vi "Send S&E Anotation message.vi"(2 "Send(T)":bool=TRUE, 7 "Annotation":string, 9 "error in (no error)":errorcluster, 12 "User(logged on)":string="Not Selected 1234", 13 "Elevated priority":bool) -> (6 "Loop ID out":u16, 10 "error out":errorcluster)   [LabVIEW 2011]
doc: "Put error message in the S&E Q. CAn also send if no error, debends exclusively on boolean in."
uses:
  emi Lib/System 01/0 - General/S&E reporting/Private/_emi_ S&E Message.ctl
  emi Lib/System 01/0 - General/S&E reporting/Private/_emi_ S&E Message type.ctl
  S&E Anotationtype.ctl
  emi Lib/System 01/0 - General/Private/_emi_GFV System ID.vi
panel:
  in  "Loc Sub ID":u16
  in  "Loop ID in(No Loop)":u16=9999
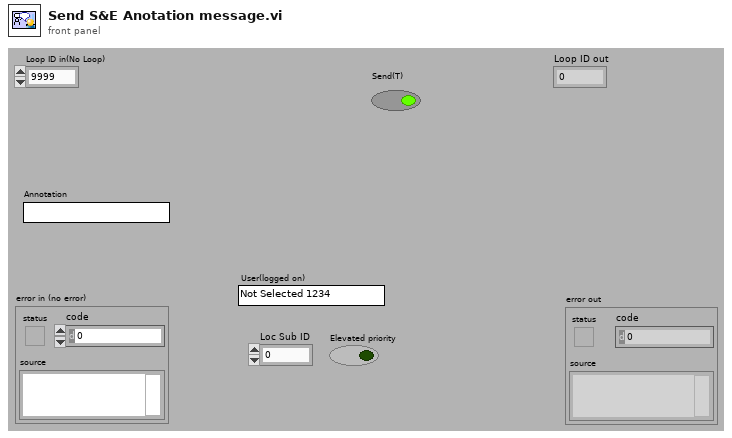
[diagram p1: front panel]
types:
  T1 = typedef "S&E Anotationtype.ctl" = cluster{"User":string, "Annotation":string}
  T2 = typedef "_emi_ S&E Message type.ctl" = enum16{"Error/Warning", "Note", "Debug", "Event", "Alarm Analog", "Alarm Digital", "Annotation"}
  T3 = typedef "_emi_ S&E Message.ctl" = cluster{"Type":T2, "Originate time":dbl, "System":u8, "Loop":u16, "Sub ID":u16, "Elevated priority":bool, "E&S Message content":variant}
  T4 = typedef "User Indikator.ctl" = cluster{"User Name":string, "Super User":T5}
  T5 = typedef "Super User bool indikator.ctl" = bool
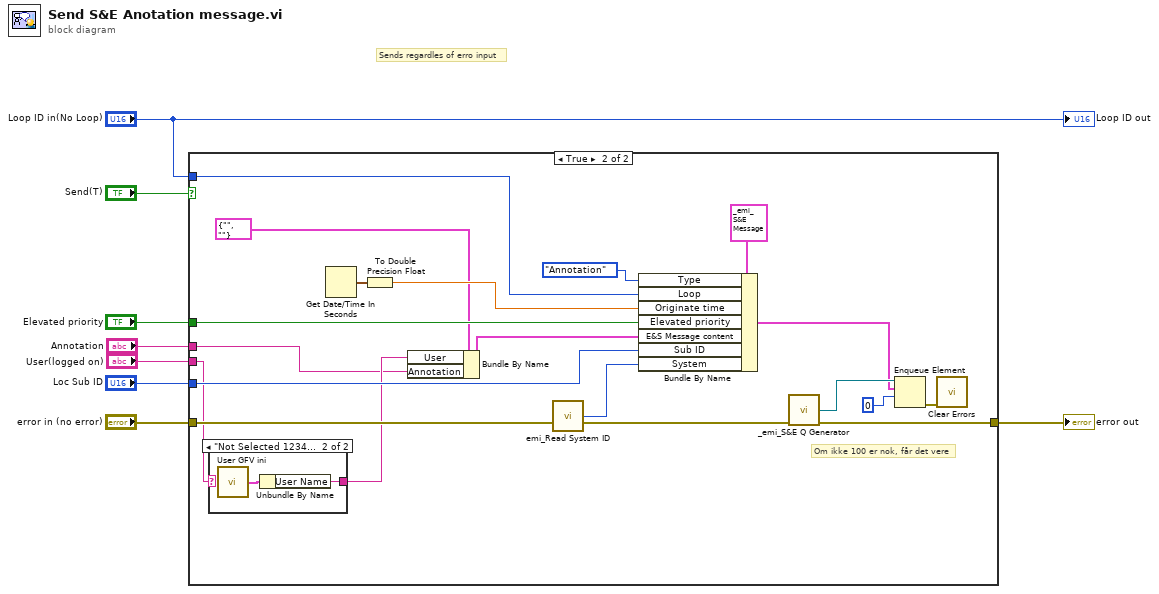
[diagram p0: block diagram]
diagram:
  # "Sends regardles of erro input"
  n1 = case shown="True" "Send(T)" {
    tunnel: "Loop ID in(No Loop)" -> [_ w25]
    tunnel: "Elevated priority" -> [_ w26]
    tunnel: "error in (no error)" -> [w9 w17]
    tunnel: [w9 w23] -> w5
    tunnel: "Loc Sub ID" -> [_ w19]
    tunnel: "User(logged on)" -> [_ w14]
    tunnel: "Annotation" -> [_ w10]
    frame False {
    }
    frame True {
      # "Om ikke 100 er nok, får det vere"
      n2 = case shown="\"Not Selected 1234\"" w14 {
        selector: w14 -> [w30 _]
        tunnel: [w30 w31] -> w11
        frame "False", Default {
        }
        frame "Not Selected 1234" {
          n3 = call "User GFV ini.vi"() -> ("User ID out"=w32:T4)  [unwired: 14 in, 1 out]
          n4 = Unbundle By Name(w32) -> ("User Name"=w31:string)
        }
      }
      n5 = Get Date/Time In Seconds() -> (seconds since 1Jan1904=w27:timestamp)
      n6 = To Double Precision Float(number=w27) -> (double precision float=w28:dbl)
      n7 = Bundle By Name(cluster=T1 {"User"="", "Annotation"=""} ("S&E Annotation"), "User"=w11, "Annotation"=w10) -> (w12:T1)
      n8 = call "emi_Read System ID.vi"("error in (no error)"=w17) -> ("System ID"=w15:u8, "error out"=w16:errorcluster)  [unwired: 13 in]
      n9 = Bundle By Name(cluster=T3 {"Type"=enum."Error/Warning", "Originate time"=0.0, "System"=0, "Loop"=0, "Sub ID"=0, "Elevated priority"=FALSE, "E&S Message content"=variant} ("E&S Message"), "Type"=_emi__S&E_Message_type."Annotation", "Loop"=w25, "Originate time"=w28, "Elevated priority"=w26, "E&S Message content"=w12, "Sub ID"=w19, "System"=w15) -> (w21:T3)
      n10 = call "_emi_S&E Q Generator.vi"("error in (no error)"=w16) -> ("E&S Message Q"=w22:refnum<queue>, "error out"=w23:errorcluster)  [unwired: 13 in]
      n11 = Enqueue Element(queue=w22, element=w21, timeout in ms (-1)=0) -> (error out=w18:errorcluster)  [unwired: 1 in, 2 out]
      n12 = call <vilib>:"Clear Errors.vi"("error in (no error)"=w18) -> ()  [unwired: 6 in, 1 out]
    }
  }
  "error out" <- w5
  "Loop ID out" <- "Loop ID in(No Loop)"
